vi "Query Headers and Data from VASP DB.vi"(8 "error in (no error)":errorcluster, 10 "Full Path":path, 11 "connection reference":T1) -> (0 "error out":errorcluster, 1 "Data":string[](array[string]), 2 "Headers":string[](array[string]), 3 "connection reference out":T1)   [LabVIEW 2010]
uses:
  <vilib>/addons/database/Connection.llb/Conn ObjectReference.ctl
  <vilib>/addons/database/_DB Variant To Data/Database Variant To Data.xnode
  <vilib>/addons/database/Connection.llb/Conn Execute.vi
  <vilib>/addons/database/Recordset.llb/Rec Fetch Recordset Data (R).vi
  <vilib>/addons/database/Recordset.llb/Rec Destroy - Connection.vi
  <vilib>/addons/database/NI_Database_API.lvlib
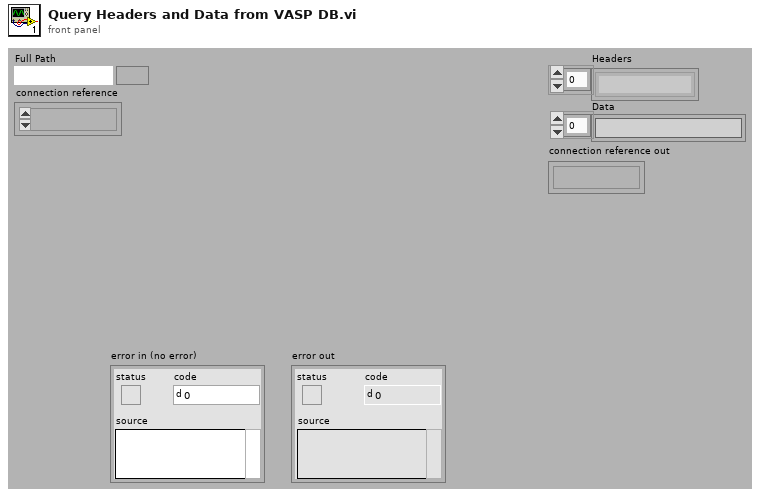
[diagram p1: front panel]
types:
  T1 = typedef "NI_Database_API.lvlib/Conn ObjectReference.ctl" = refnum<k1>
  T2 = typedef "NI_Database_API.lvlib/Rec ObjectReference.ctl" = refnum<k1>
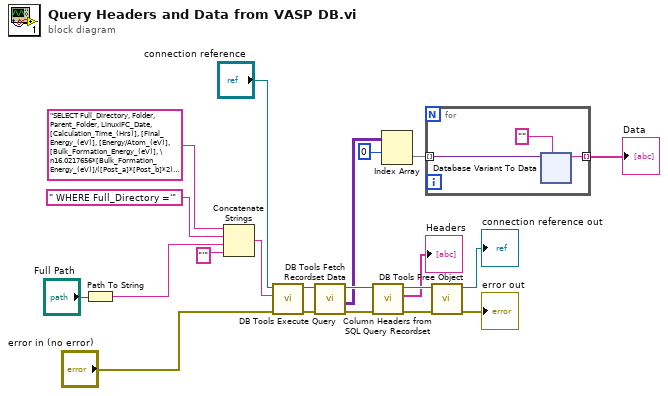
[diagram p0: block diagram]
diagram:
  n1 = Path To String(path="Full Path") -> (string=w19:string)
  n2 = Concatenate Strings("SELECT Full_Directory, Folder, Parent_Folder, LinuxIFC_Date, [Calculation_Time_(Hrs)], [Final_Energy_(eV)], [Energy/Atom_(eV)], [Bulk_Formation_Energy_(eV)], \n16.0217656*[Bulk_Formation_Energy_(eV)]/([Post_a]*[Post_b]*2) AS [Interfacial_Energy_(J/m²)],\nIonic_Steps, Num_Atoms, Post_Structure, Post_a, Post_b, Post_c, Post_alpha, Post_beta, Post_gamma, [Ion_Motion_(IBRION)], [Degrees_of_Freedom_(ISIF)], \n[Partial_Occupancies_(ISMEAR)], [Spin_polarizaiton_(ISPIN)], Defect_Name, Location, Defect_Free_Structure_Name, Net_Charge, [Net Charge (Defect)], Comments\nFROM     Master_VASP_View", " WHERE Full_Directory ='" ("string"), w19, "'" ("string")) -> (w16:string)
  n3 = call-poly <vilib>:"DB Tools Execute Query.vi"("error in (no error)"="error in (no error)", "SQL query"=w16, "connection reference"="connection reference") -> ("error out"=w7:errorcluster, "recordset reference"=w15:T2)  [unwired: 5 in]
  n4 = call-poly <vilib>:"DB Tools Fetch Recordset Data.vi"("error in (no error)"=w7, "recordset reference"=w15) -> ("error out"=w5:errorcluster, "recordset data"=w11:variant[][], "recordset reference out"=w14:T2)  [unwired: 3 in]
  n5 = call "Column Headers from SQL Query Recordset.vi"("error in (no error)"=w5, "recordset reference"=w14) -> ("error out"=w6:errorcluster, "columns"=→"Headers":string[], "Recordset reference Out"=w13:T2)  [unwired: 6 in, 1 out]
  n6 = Index Array(array=w11, index (row)=0) -> (element=w9:variant[])  [unwired: 1 in]
  n7 = for {
    tunnel: w9 -> [w24] mode=indexing
    tunnel: [w22] -> w8 mode=indexing
    n8 = xnode "Database Variant To Data"("database variant"=w24, "type"="") -> ("data"=w22:string)  [unwired: 1 in, 1 out]
  }
  "Data" <- w8
  n9 = call-poly <vilib>:"DB Tools Free Object.vi"("error in (no error)"=w6, "recordset reference"=w13) -> ("error out"=→"error out":errorcluster, "connection reference"=→"connection reference out":T1)  [unwired: 8 in]
